vi "PH_AWG-510.Evt Call Start Device.vi"(0 "i ref in":refnum<vi>, 1 "Instance":string, 2 "Start Device":bool, 5 "error in":errorcluster) -> (14 "i ref out":refnum<vi>, 19 "error out":errorcluster)   [LabVIEW 2014, in "PH_AWG-510.lvlib"]
doc: "This VI calls a method by a simple call."
uses:
  CSCore/CSSystem/CoreLib/CoreLib.short 2 byte array.vi
  PH_AWG-510.lvlib
  CSCore/CSSystem/CoreLib/CoreLib.lvlib
  CSCore/BaseProcess/BaseProcess.lvlib
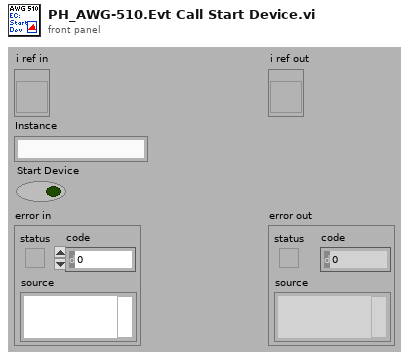
[diagram p1: front panel]
types:
  T1 = typedef "CoreDefs.rawDataType.ctl" = i8[]
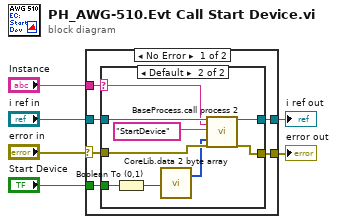
[diagram p0: block diagram]
diagram:
  n1 = case shown="No Error" "error in" {
    selector: "error in" -> [w9 w24]
    tunnel: [w12 w24] -> w3
    tunnel: "Instance" -> [w8 _]
    tunnel: "i ref in" -> [w11 w25]
    tunnel: [w10 w25] -> w5
    tunnel: "Start Device" -> [w7 _]
    frame No Error {
      n2 = case shown="Default" w8 {
        selector: w8 -> [_ w17]
        tunnel: [w14 w23] -> w12
        tunnel: w9 -> [w14 w21]
        tunnel: w11 -> [w13 w20]
        tunnel: [w13 w19] -> w10
        tunnel: w7 -> [_ w16]
        frame "", "N/A" {
        }
        frame Default {
          n3 = Boolean To (0,1)(Boolean=w16) -> (0, 1=w15:i16)
          n4 = call-poly "CoreLib.data 2 byte array.vi"("i16"=w15) -> ("byteArray out"=w18:T1)  [unwired: 18 in]
          n5 = call "BaseProcess.call process 2.vi"("i ref in"=w20, "Object"=w17, "Selector"="StartDevice", "Data"=w18, "error in (no error)"=w21) -> ("i ref out"=w19:refnum<vi>, "error out"=w23:errorcluster)  [unwired: 13 in]
        }
      }
    }
    frame Error {
    }
  }
  "i ref out" <- w5
  "error out" <- w3
